vi "Schedule.vi"(7 "Choice":i32=-1, 11 "Blueprint in":refnum<class "Blueprint.lvclass">) -> (1 "Finished?":bool, 2 "# elements in queue":i32, 3 "Blueprint out":refnum<class "Blueprint.lvclass">)   [LabVIEW 2023, in "d19.lvlib" / "Blueprint.lvclass"]
uses:
  Blueprint/Blueprint.lvclass
  Blueprint/Blueprint.lvclass/Blueprint.ctl
  Mine/Mine.lvclass
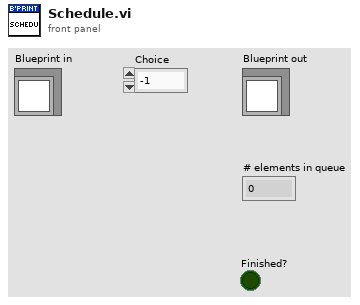
[diagram p1: front panel]
types:
  T1 = cluster{"Ore Robot Ore Cost":u8, "Clay Robot Ore Cost":u8, "Obsidian Robot Ore Cost":u8, "Geode Robot Ore Cost":u8, "Obsidian Robot Clay Cost":u8, "Geode Robot Obsidian Cost":u8}
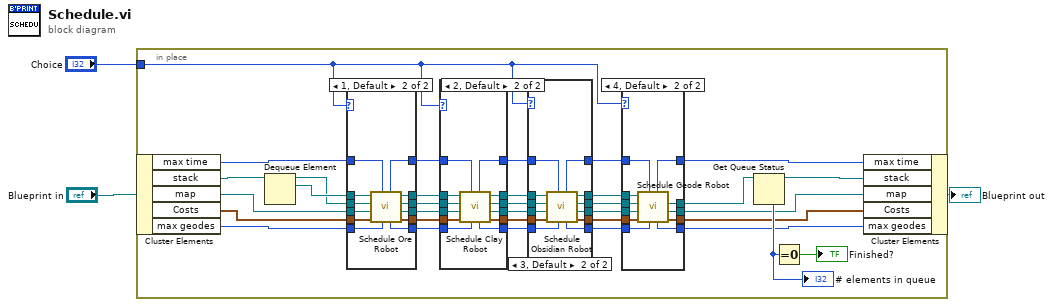
[diagram p0: block diagram]
diagram:
  n1 = in-place {
    in-place-border: "Choice" -> [w10]
    n2 = in-place-cluster #1("Blueprint in") -> ("max time"=w11:u8, "stack"=w17:refnum<queue>, "map"=w7:refnum<data-value>, "Costs"=w6:T1, "max geodes"=w5:u8)
    n3 = Dequeue Element(queue=w17) -> (queue out=w8:refnum<queue>, element=w9:refnum<class "Mine.lvclass">)  [unwired: 2 in, 2 out]
    n4 = case shown="1, Default" w10 {
      tunnel: [w95 w107] -> w24
      tunnel: [w94 w106] -> w23
      tunnel: w8 -> [w93 w105]
      tunnel: [w93 w104] -> w22
      tunnel: [w91 w103] -> w21
      tunnel: [w90 w102] -> w20
      tunnel: w9 -> [w94 w101]
      tunnel: [w92 w100] -> w19
      tunnel: w11 -> [w95 w99]
      tunnel: w6 -> [w91 w98]
      tunnel: w7 -> [w92 w97]
      tunnel: w5 -> [w90 w96]
      frame 2..4 {
      }
      frame 1, Default {
        n5 = call "Schedule Ore Robot.vi"("max geodes in"=w96, "max time in"=w99, "costs in"=w98, "data value reference"=w97, "stack in"=w105, "mine in"=w101) -> ("costs out"=w103:T1, "data value reference"=w100:refnum<data-value>, "stack out"=w104:refnum<queue>, "mine out"=w106:refnum<class "Mine.lvclass">, "max geodes out"=w102:u8, "max time out"=w107:u8)
      }
    }
    n6 = case shown="2, Default" w10 {
      tunnel: [w76 w89] -> w30
      tunnel: [w77 w88] -> w29
      tunnel: [w75 w87] -> w28
      tunnel: [w74 w86] -> w27
      tunnel: [w73 w85] -> w26
      tunnel: [w72 w84] -> w25
      tunnel: w24 -> [w77 w83]
      tunnel: w23 -> [w76 w82]
      tunnel: w22 -> [w75 w81]
      tunnel: w21 -> [w73 w80]
      tunnel: w20 -> [w72 w79]
      tunnel: w19 -> [w74 w78]
      frame 1, 3, 4 {
      }
      frame 2, Default {
        n7 = call "Schedule Clay Robot.vi"("max geodes in"=w79, "max time in"=w83, "costs in"=w80, "data value reference"=w78, "stack in"=w81, "mine in"=w82) -> ("costs out"=w85:T1, "data value reference"=w86:refnum<data-value>, "stack out"=w87:refnum<queue>, "mine out"=w89:refnum<class "Mine.lvclass">, "max geodes out"=w84:u8, "max time out"=w88:u8)
      }
    }
    n8 = case shown="3, Default" w10 {
      tunnel: [w59 w71] -> w36
      tunnel: [w58 w70] -> w35
      tunnel: [w57 w69] -> w34
      tunnel: [w56 w68] -> w33
      tunnel: [w55 w67] -> w32
      tunnel: [w54 w66] -> w31
      tunnel: w30 -> [w58 w65]
      tunnel: w29 -> [w59 w64]
      tunnel: w28 -> [w57 w63]
      tunnel: w27 -> [w56 w62]
      tunnel: w26 -> [w55 w61]
      tunnel: w25 -> [w54 w60]
      frame 1, 2, 4 {
      }
      frame 3, Default {
        n9 = call "Schedule Obsidian Robot.vi"("max geodes in"=w60, "max time in"=w64, "costs in"=w61, "data value reference"=w62, "stack in"=w63, "mine in"=w65) -> ("costs out"=w67:T1, "data value reference"=w68:refnum<data-value>, "stack out"=w69:refnum<queue>, "mine out"=w70:refnum<class "Mine.lvclass">, "max geodes out"=w66:u8, "max time out"=w71:u8)
      }
    }
    n10 = case shown="4, Default" w10 {
      tunnel: w36 -> [w42 w53]
      tunnel: w35 -> [_ w52]
      tunnel: w34 -> [w41 w51]
      tunnel: w33 -> [w40 w50]
      tunnel: w32 -> [w39 w49]
      tunnel: w31 -> [w38 w48]
      tunnel: [w42 w47] -> w18
      tunnel: [w38 w46] -> w16
      tunnel: [w41 w45] -> w15
      tunnel: [w40 w44] -> w13
      tunnel: [w39 w43] -> w12
      frame 1..3 {
      }
      frame 4, Default {
        n11 = call "Schedule Geode Robot.vi"("max geodes in"=w48, "max time in"=w53, "costs in"=w49, "data value reference"=w50, "stack in"=w51, "mine in"=w52) -> ("costs out"=w43:T1, "data value reference"=w44:refnum<data-value>, "stack out"=w45:refnum<queue>, "max geodes out"=w46:u8, "max time out"=w47:u8)  [unwired: 1 out]
      }
    }
    n12 = Get Queue Status(queue=w15) -> (queue out=w14:refnum<queue>, # elements in queue=w37:i32)  [unwired: 2 in, 6 out]
    "# elements in queue" <- w37
    n13 = Equal To 0?(x=w37) -> (x = 0?=→"Finished?":bool)
    n14 = in-place-cluster #1("max time"=w18, "stack"=w14, "map"=w13, "Costs"=w12, "max geodes"=w16) -> (→"Blueprint out":refnum<class "Blueprint.lvclass">)
  }
